vi "Settings.Create.vi"(8 "error in (no error)":errorcluster, 10 "Settings Channels":T2[](array[typedef]), 11 "Section Ref in":T1 format="%.0x") -> (0 "error out":errorcluster, 3 "nodeID out":u64)   [LabVIEW 2019, in "Diagnostics Addon Shared.lvlib"]
uses:
  Diagnostics Addon Shared.lvlib
  Types/Settings.Channel.ctl
  <vilib>/NI VeriStand/Custom Device API/Custom Device Channel.ctl
  <vilib>/NI VeriStand/Custom Device API/Custom Device Channel Type.ctl
  <vilib>/NI VeriStand/Custom Device API/Custom Device Item Ref.ctl
  Constants.vi
  <vilib>/NI/NI VeriStand Advanced SysDef API/SysDef API/Advanced System Definition.lvlib
  <vilib>/NI VeriStand/Custom Device API/Custom Device API.lvlib
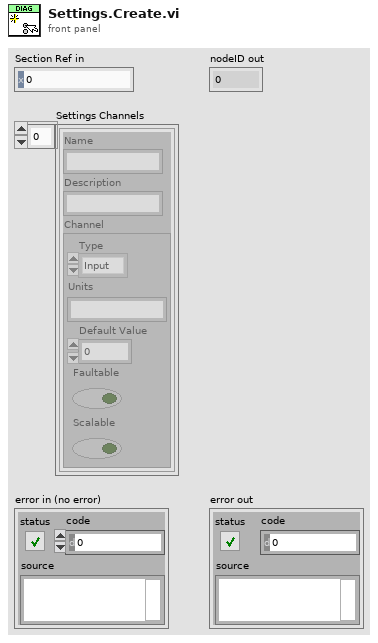
[diagram p1: front panel]
types:
  T1 = typedef "Custom Device API.lvlib/Custom Device Item Ref.ctl" = u64
  T2 = typedef "Diagnostics Addon Shared.lvlib/Settings.Channel.ctl" = cluster{"Name":string, "Description":string, "Channel":T3}
  T3 = typedef "Custom Device API.lvlib/Custom Device Channel.ctl" = cluster{"Type":T4, "Units":string, "Default Value":dbl, "Faultable":bool, "Scalable":bool}
  T4 = typedef "Custom Device API.lvlib/Custom Device Channel Type.ctl" = enum16{"Input", "Output"}
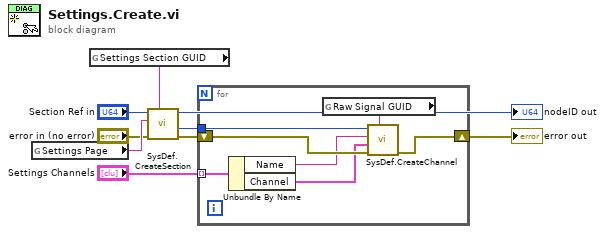
[diagram p0: block diagram]
diagram:
  n1 = global read "Constants.vi" "Settings Page"() -> (w9:string)
  n2 = global read "Constants.vi" "Settings Section GUID"() -> (w8:string)
  n3 = call <vilib>:"SysDef.CreateSection.vi"("GUID"=w8, "error in (no error)"="error in (no error)", "Name"=w9, "nodeID"="Section Ref in") -> ("error out"=w3:errorcluster, "New NodeID"=w4:u64, "nodeID out"=→"nodeID out":u64)  [unwired: 4 in, 1 out]
  n4 = for {
    tunnel: w4 -> [w14]
    shift-right: [w13] -> w5
    shift-left: w3 -> [w15]
    tunnel: "Settings Channels" -> [w12] mode=indexing
    n5 = Unbundle By Name(w12) -> ("Name"=w11:string, "Channel"=w10:T3)
    n6 = global read "Constants.vi" "Raw Signal GUID"() -> (w16:string)
    n7 = call <vilib>:"SysDef.CreateChannel.vi"("GUID"=w16, "error in (no error)"=w15, "Channel"=w10, "Name"=w11, "nodeID"=w14) -> ("error out"=w13:errorcluster)  [unwired: 3 in, 3 out]
  }
  "error out" <- w5
